vi "heatmap_lines.vi"() -> ()   [LabVIEW 2015]
uses:
  <vilib>/Utility/file.llb/Read Delimited Spreadsheet (DBL).vi
panel:
  out "Intensity Graph 2":dbl[][](graph)
  out "all rows 2":dbl[](array[numeric])
  out "all rows":dbl[][](array[numeric])
  in  "Path":path
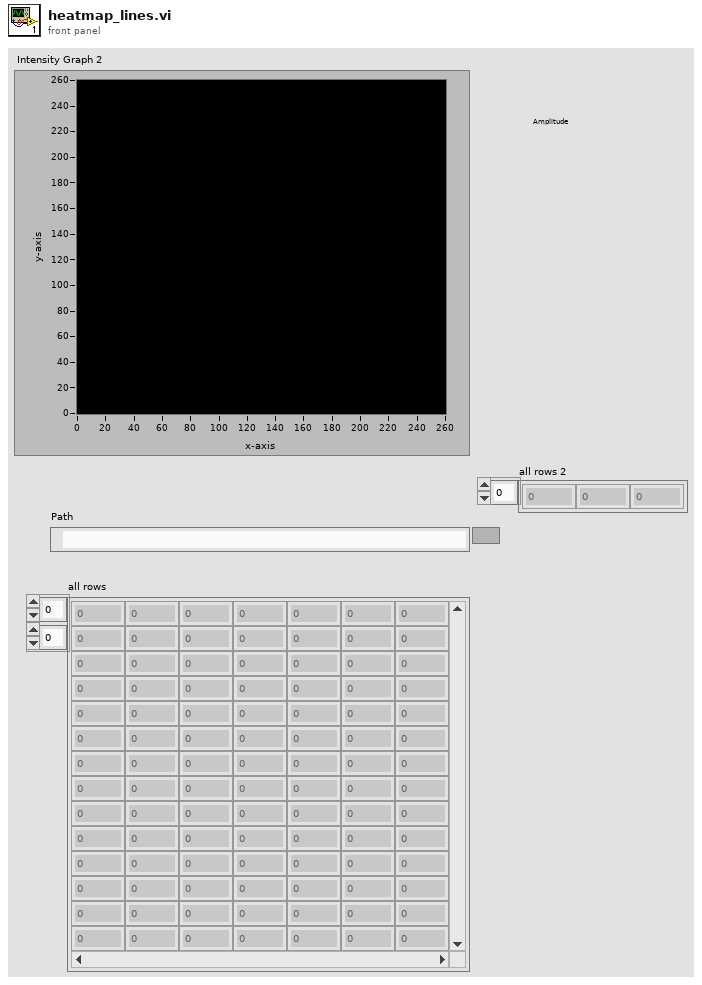
[diagram p1: front panel]
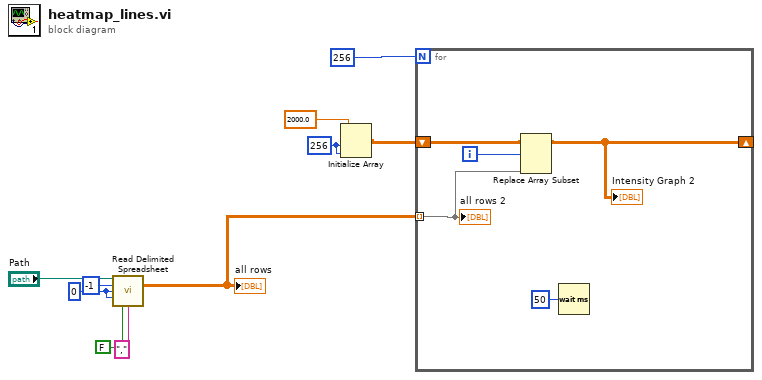
[diagram p0: block diagram]
diagram:
  w3 = 256 ("dimension size")
  w7 = 0 ("start of read offset (chars.:0)")
  n1 = call-poly <vilib>:"Read Delimited Spreadsheet.vi"("file path (dialog if empty)"="Path", "number of rows (all:-1)"=-1, "start of read offset (chars.:0)"=w7, "max characters/row  (no limit:0)"=w7, "transpose? (F)"=FALSE, "delimiter (\\t)"="," ("delimiter (\\t)")) -> ("all rows"=w4:dbl[][])  [unwired: 4 in, 5 out]
  "all rows" <- w4
  n2 = Initialize Array(2000.0 ("element"), w3, w3) -> (w1:dbl[][])
  n3 = for {
    N: 256 -> [_]
    tunnel: w4 -> [w11] mode=indexing
    shift-right: [w14] -> _
    shift-left: w1 -> [w13]
    i -> [w12]
    n4 = Replace Array Subset(array=w13, new element=w11, index (row)=w12) -> (w14:dbl[][])  [unwired: 1 in]
    "Intensity Graph 2" <- w14
    n5 = Wait (ms)(milliseconds to wait=u32 50) -> ()  [unwired: 1 out]
    "all rows 2" <- w11
  }
